vi "LHF.DB.Mongo.Bson.ToVariant.vi"(7 "type":variant, 8 "error in (no error)":errorcluster, 11 "BsonValue":refnum<k24>) -> (0 "error out":errorcluster, 2 "data":variant, 3 "BsonValue 2":refnum<k24>)   [LabVIEW 2013, in "LHF.DB.Mongo.lvclass"]
uses:
  LHF.DB.Mongo.lvclass
  C:/Users/Ricardo/Desktop/Projetos/LabVIEW-MongoDB/src/Driver/MongoDB.Bson.dll
  Driver/MongoDB.Bson.dll
  <vilib>/Utility/VariantDataType/VariantType.lvlib
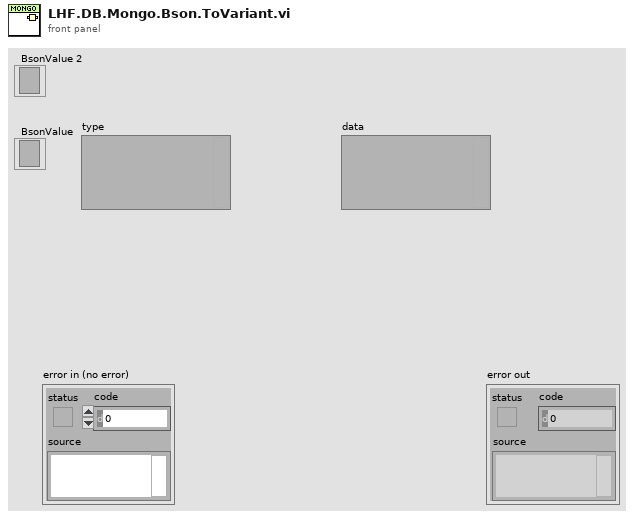
[diagram p1: front panel]
types:
  T1 = typedef "VariantType.lvlib/Type.ctl" = enum8{"Invalid Type", "Void", "I8", "I16", "I32", "I64", "U8", "U16", "U32", "U64", "Single Float", "Double Float", "Extended Float", "Single Complex", "Double Complex", "Extended Complex", "Enum U8", "Enum U16", "Enum U32", "Enum U64", "Single Float With Unit", "Double Float With Unit", "Extended Float With Unit", "Single Complex with Unit", "Double Complex with Unit", "Extended Complex with Unit", "Boolean", "String", "Path", "Picture", "Tag", "Array", "Cluster", "Variant", "LV Variant", "Waveform", "Timestamp", "Digital Waveform", "Digital Data", "ExpressData", "Refnum", "External Data", "VI", "Poly VI", "LabVIEW Class Instance", "Fixed Point"}
  T2 = typedef "LHF.DB.Mongo.lvclass/LHF.DB.Mongo.Typedef.VariantData.ctl" = cluster{"Type Enum":T1, "Name":string, "Variant":variant}
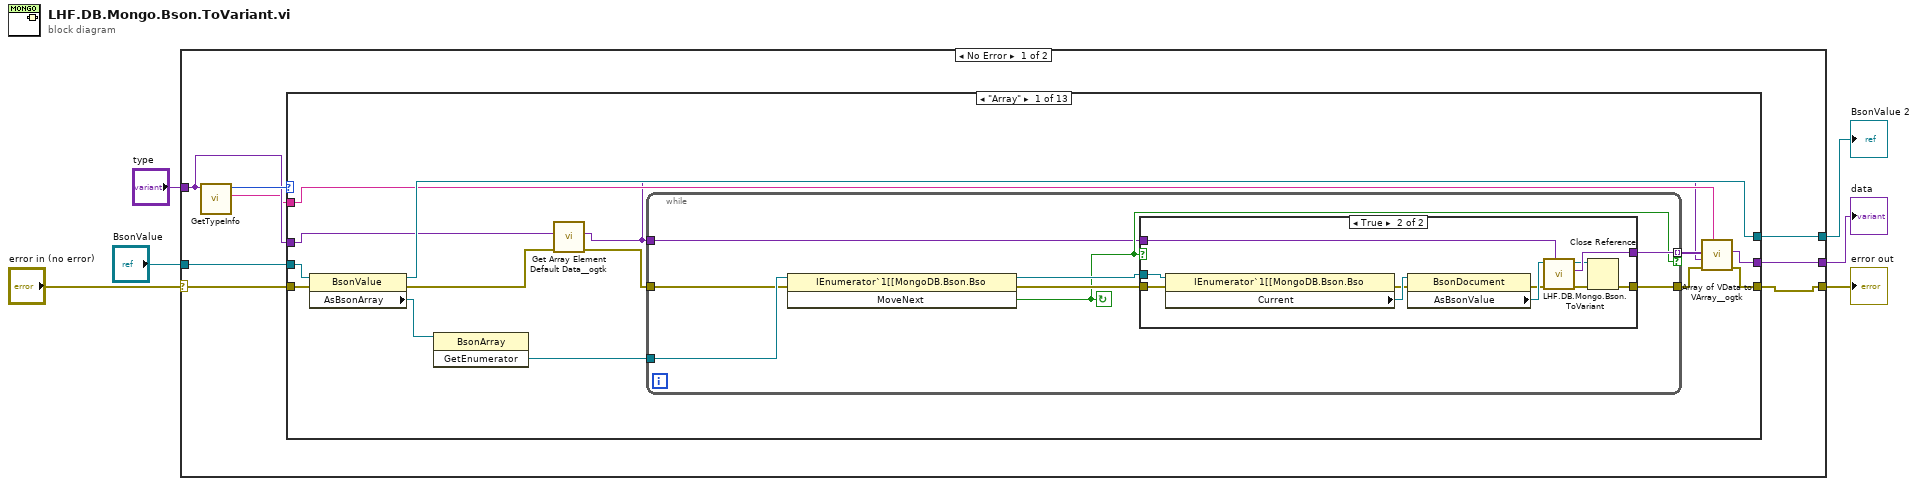
[diagram p0: block diagram]
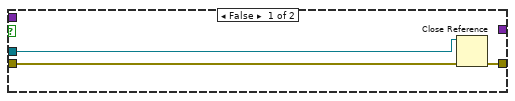
[diagram p2: hidden frame]
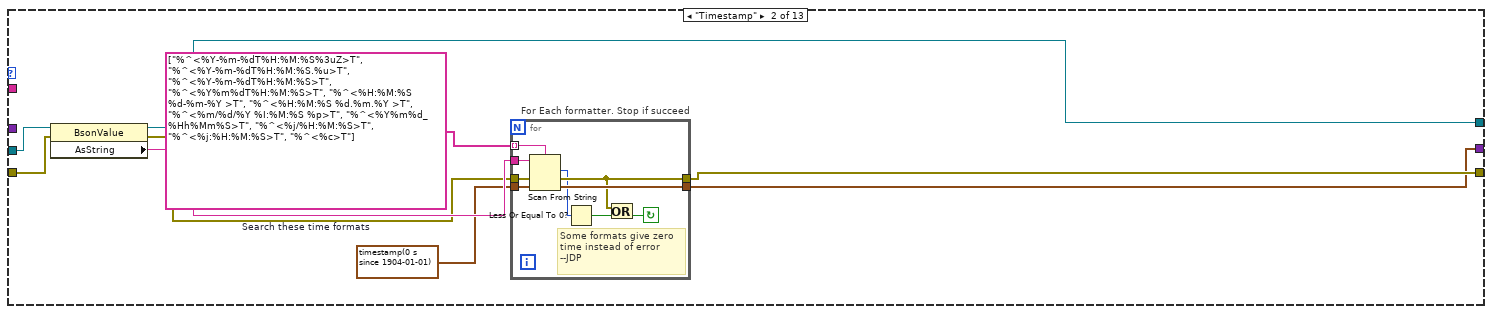
[diagram p3: hidden frame]
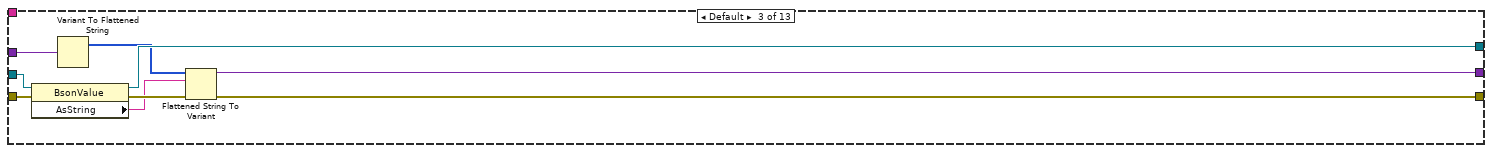
[diagram p4: hidden frame]
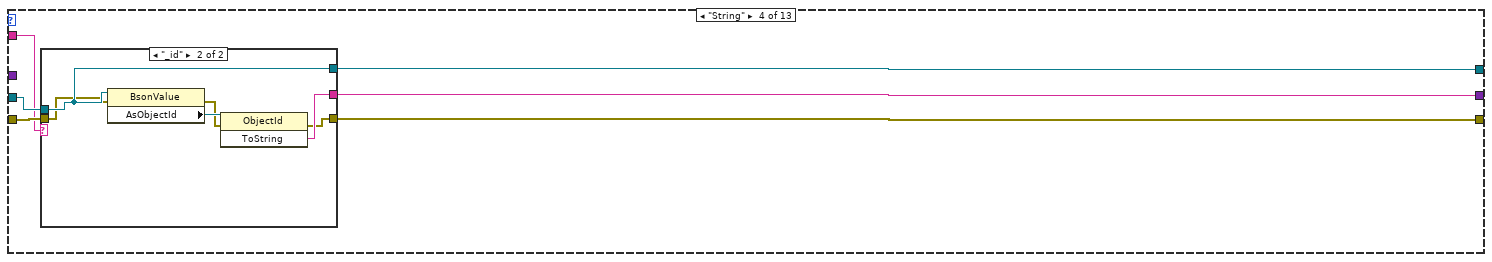
[diagram p5: hidden frame]
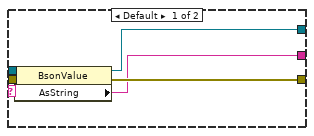
[diagram p6: hidden frame]
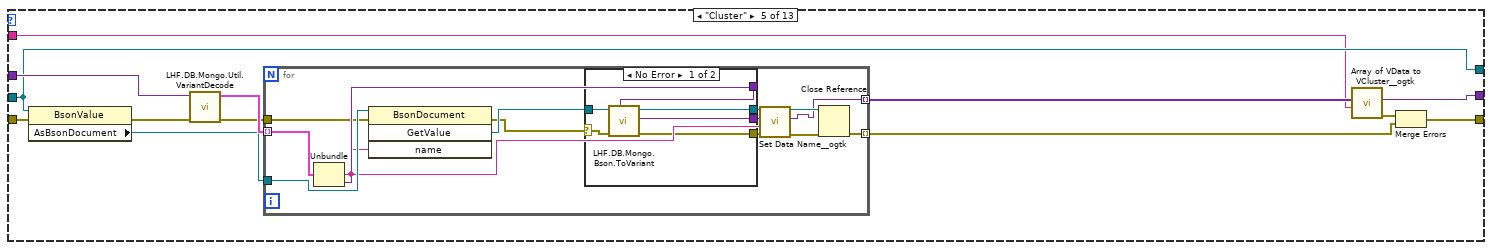
[diagram p7: hidden frame]
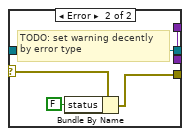
[diagram p8: hidden frame]
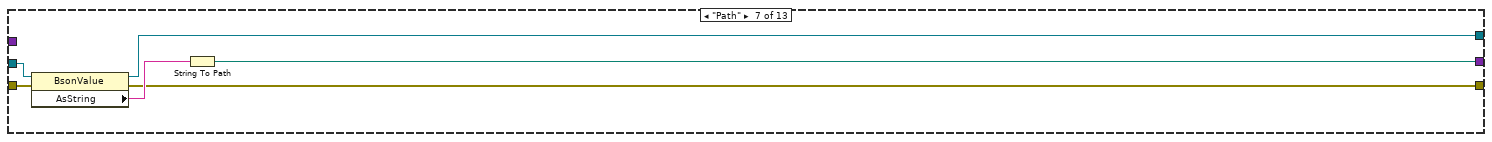
[diagram p10: hidden frame]
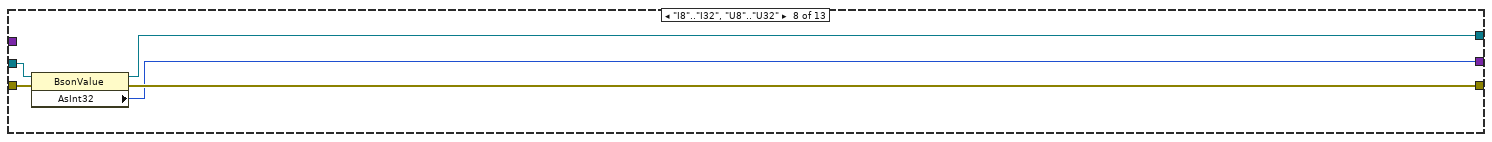
[diagram p11: hidden frame]
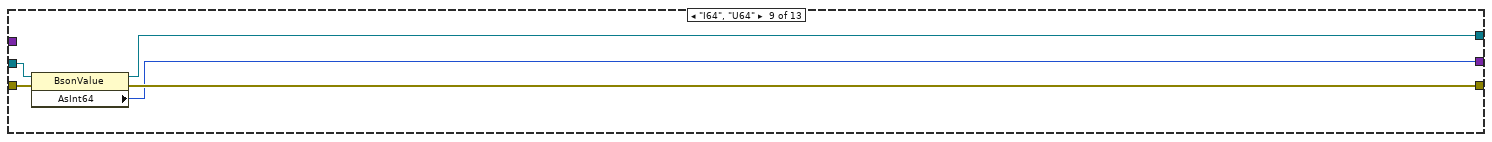
[diagram p12: hidden frame]
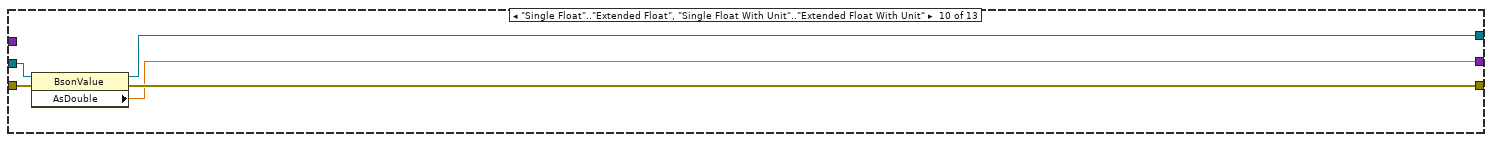
[diagram p13: hidden frame]
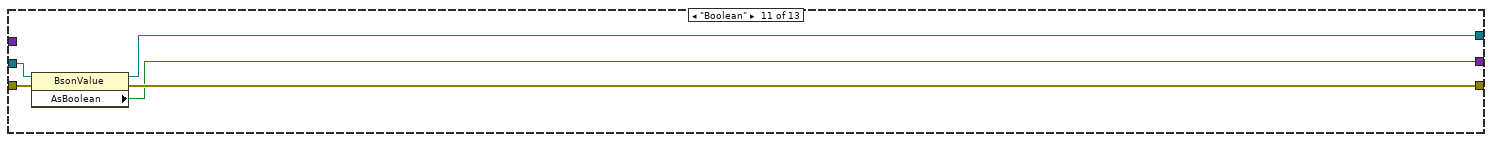
[diagram p14: hidden frame]
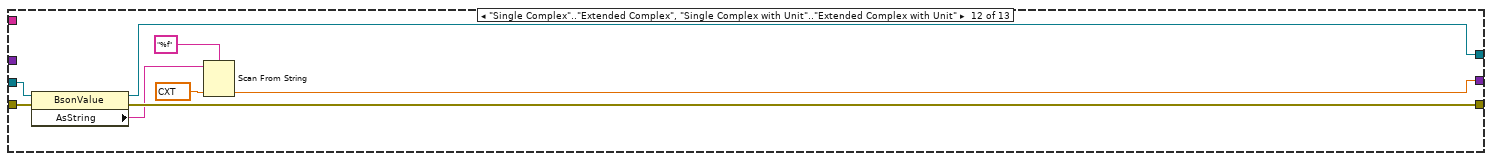
[diagram p15: hidden frame]
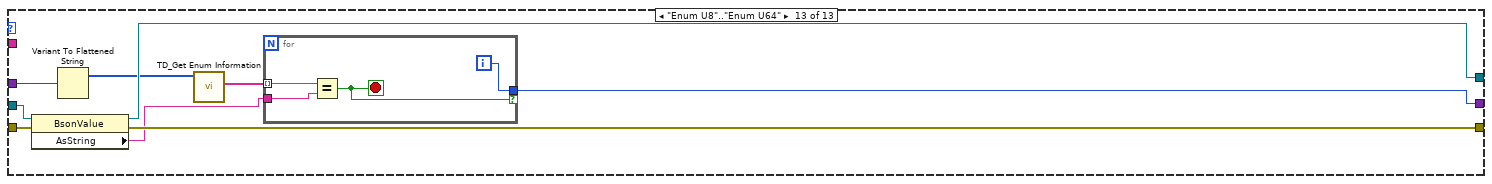
[diagram p16: hidden frame]
diagram:
  n1 = case shown="No Error" "error in (no error)" {
    selector: "error in (no error)" -> [w12 w183]
    tunnel: [w8 w183] -> w5
    tunnel: "BsonValue" -> [w14 w182]
    tunnel: "type" -> [w10 _]
    tunnel: [w13 w182] -> w2
    tunnel: [w7 _] -> w1
    frame No Error {
      n2 = call <vilib>:"GetTypeInfo.vi"("Variant"=w10) -> ("Name"=w9:string, "Type Enum"=w11:T1)  [unwired: 6 in, 3 out]
      n3 = case shown="\"Array\"" w11 {
        tunnel: w14 -> [w28 w58 w77 w83 w100 w133 w140 w145 w150 w155 w160 w168 w177]
        tunnel: [w26 w52 w75 w81 w100 w133 w136 w142 w147 w152 w157 w165 w174] -> w13
        tunnel: [w18 w51 w69 w79 w99 w134 w135 w141 w146 w151 w156 w162 w169] -> w7
        tunnel: w12 -> [w27 w54 w76 w82 w97 w132 w138 w144 w149 w154 w159 w167 w176]
        tunnel: [w15 w53 w71 w80 w103 w132 w137 w143 w148 w153 w158 w166 w175] -> w8
        tunnel: w10 -> [w23 _ w74 _ w107 w134 _ _ _ _ _ _ w173]
        tunnel: w9 -> [w17 _ _ w78 w95 _ _ _ _ _ _ _ _]
        frame "Array" {
          n4 = property class="BsonValue"(reference=w28, error in=w27) -> (reference out=w26:refnum<k24>, error out=w22:errorcluster, "AsBsonArray"=w25:refnum<k24>)
          n5 = invoke class="BsonArray" method="GetEnumerator"(reference=w25) -> ("GetEnumerator"=w24:refnum<k24>)  [unwired: 2 in, 2 out]
          n6 = call <userlib>:"Get Array Element Default Data__ogtk.vi"("error in (no error)"=w22, "Array"=w23) -> ("error out"=w21:errorcluster, "Array Element Default Data"=w16:variant)  [unwired: 8 in]
          n7 = while {
            tunnel: [w34] -> w19 mode=indexing if=w31
            tunnel: [w32] -> w20
            tunnel: w24 -> [w36]
            tunnel: w16 -> [w30]
            tunnel: w21 -> [w29]
            stop <- w31 continue-if-true
            n8 = invoke class="IEnumerator`1[[MongoDB.Bson.Bso" method="MoveNext"(reference=w36, error in=w29) -> (reference out=w35:refnum<k24>, error out=w33:errorcluster, "MoveNext"=w31:bool)  [unwired: 1 in]
            n9 = case shown="True" w31 {
              tunnel: w35 -> [w38 w50]
              tunnel: [_ w47] -> w34
              tunnel: w33 -> [w39 w49]
              tunnel: [w37 w48] -> w32
              tunnel: w30 -> [_ w46]
              frame False {
                n10 = Close Reference(reference=w38, error in (no error)=w39) -> (error out=w37:errorcluster)
              }
              frame True {
                n11 = property class="IEnumerator`1[[MongoDB.Bson.Bso"(reference=w50, error in=w49) -> (error out=w41:errorcluster, "Current"=w43:refnum<k24>)  [unwired: 1 out]
                n12 = property class="BsonDocument"(reference=w43, error in=w41) -> (error out=w40:errorcluster, "AsBsonValue"=w42:refnum<k24>)  [unwired: 1 out]
                n13 = call "LHF.DB.Mongo.Bson.ToVariant.vi"("type"=w46, "error in (no error)"=w40, "BsonValue"=w42) -> ("error out"=w44:errorcluster, "data"=w47:variant, "BsonValue 2"=w45:refnum<k24>)  [unwired: 6 in]
                n14 = Close Reference(reference=w45, error in (no error)=w44) -> (error out=w48:errorcluster)
              }
            }
          }
          n15 = call <userlib>:"Array of VData to VArray__ogtk.vi"("Array Name"=w17, "error in (no error)"=w20, "Element Type (when empty)"=w16, "1D Array of VData"=w19) -> ("error out"=w15:errorcluster, "VArray"=w18:variant)  [unwired: 6 in]
        }
        frame "Timestamp" {
          w59 = string[] ["%^<%Y-%m-%dT%H:%M:%S%3uZ>T", "%^<%Y-%m-%dT%H:%M:%S.%u>T", "%^<%Y-%m-%dT%H:%M:%S>T", "%^<%Y%m%dT%H:%M:%S>T", "%^<%H:%M:%S %d-%m-%Y >T", "%^<%H:%M:%S %d.%m.%Y >T", "%^<%m/%d/%Y %I:%M:%S %p>T", "%^<%Y%m%d_%Hh%Mm%S>T", "%^<%j/%H:%M:%S>T", "%^<%j:%H:%M:%S>T", "%^<%c>T"]  # Search these time formats
          n16 = property class="BsonValue"(reference=w58, error in=w54) -> (reference out=w52:refnum<k24>, error out=w55:errorcluster, "AsString"=w57:string)
          n17 = for "For Each formatter. Stop if succeed" {
            tunnel: [w68] -> w51
            tunnel: w55 -> [w67]
            tunnel: [w61] -> w53
            tunnel: timestamp(0 s since 1904-01-01) ("default value 1") -> [w66]
            tunnel: w57 -> [w65]
            tunnel: w59 -> [w64] mode=indexing
            stop <- w62 continue-if-true
            # "Some formats give zero\ntime instead of error\n--JDP"
            n18 = Scan From String(format string=w64, input string=w65, error in=w67, default 1=w66) -> (offset past scan=w60:u32, error out=w61:errorcluster, output 1=w68:timestamp)  [unwired: 1 in, 1 out]
            n19 = Less Or Equal To 0?(x=w60) -> (x <= 0?=w63:bool)
            n20 = Or(x=w61, y=w63) -> (x .or. y?=w62:bool)
          }
        }
        frame Default {
          n21 = property class="BsonValue"(reference=w77, error in=w76) -> (reference out=w75:refnum<k24>, error out=w72:errorcluster, "AsString"=w70:string)
          n22 = Variant To Flattened String(Variant=w74) -> (1:w73:i16[])  [unwired: 1 out]
          n23 = Flattened String To Variant(4:w72, 6:w70, 7:w73) -> (0:w71:errorcluster, 3:w69:variant)
        }
        frame "String" {
          n24 = case shown="\"_id\"" w78 {
            tunnel: w83 -> [w88 w92]
            tunnel: w82 -> [w87 w89]
            tunnel: [w86 w92] -> w81
            tunnel: [w85 w91] -> w80
            tunnel: [w84 w93] -> w79
            frame Default {
              n25 = property class="BsonValue"(reference=w88, error in=w87) -> (reference out=w86:refnum<k24>, error out=w85:errorcluster, "AsString"=w84:string)
            }
            frame "_id" {
              n26 = property class="BsonValue"(reference=w92, error in=w89) -> (error out=w90:errorcluster, "AsObjectId"=w94:refnum<k24>)  [unwired: 1 out]
              n27 = invoke class="ObjectId" method="ToString"(reference=w94, error in=w90) -> (error out=w91:errorcluster, "ToString"=w93:string)  [unwired: 1 in, 1 out]
            }
          }
        }
        frame "Cluster" {
          n28 = property class="BsonValue"(reference=w100, error in=w97) -> (error out=w102:errorcluster, "AsBsonDocument"=w96:refnum<k24>)  [unwired: 1 out]
          n29 = call "LHF.DB.Mongo.Util.VariantDecode.vi"("error in (no error)"=w102, "variant"=w107) -> ("error out"=w101:errorcluster, "Variant Data"=w106:T2[])  [unwired: 7 in, 1 out]
          n30 = for {
            tunnel: w106 -> [w120] mode=indexing
            tunnel: w96 -> [w118]
            tunnel: [w110] -> w105 mode=indexing
            tunnel: [w116] -> w104 mode=indexing
            tunnel: w101 -> [w115]
            n31 = Unbundle(w120) -> ("Name"=w112:string, "Variant"=w119:variant)  [unwired: 1 out]
            n32 = invoke class="BsonDocument" method="GetValue"(reference=w118, error in=w115, "name"=w112) -> (error out=w108:errorcluster, "GetValue"=w114:refnum<k24>)  [unwired: 1 in, 2 out]
            n33 = case shown="No Error" w108 {
              selector: w108 -> [w121 w129]
              tunnel: w119 -> [w126 w131]
              tunnel: [w125 w130] -> w117
              tunnel: w114 -> [w124 w130]
              tunnel: [w123 w128] -> w113
              tunnel: [w122 w131] -> w111
              frame No Error {
                n34 = call "LHF.DB.Mongo.Bson.ToVariant.vi"("type"=w126, "error in (no error)"=w121, "BsonValue"=w124) -> ("error out"=w123:errorcluster, "data"=w122:variant, "BsonValue 2"=w125:refnum<k24>)  [unwired: 6 in]
              }
              frame Error {
                # "TODO: set warning decently\nby error type"
                n35 = Bundle By Name(cluster=w129, "status"=FALSE) -> (w128:errorcluster)
              }
            }
            n36 = call <userlib>:"Set Data Name__ogtk.vi"("error in (no error)"=w113, "Data Name"=w112, "Data"=w111) -> ("error out"=w109:errorcluster, "Renamed Data"=w110:variant)  [unwired: 7 in]
            n37 = Close Reference(reference=w117, error in (no error)=w109) -> (error out=w116:errorcluster)
          }
          n38 = call <userlib>:"Array of VData to VCluster__ogtk.vi"("Cluster Name"=w95, "Array"=w105) -> ("error out"=w98:errorcluster, "VCluster"=w99:variant)  [unwired: 8 in]
          n39 = Merge Errors(w98, w104) -> (w103:errorcluster)
        }
        frame "Void" {
        }
        frame "Path" {
          n40 = property class="BsonValue"(reference=w140, error in=w138) -> (reference out=w136:refnum<k24>, error out=w137:errorcluster, "AsString"=w139:string)
          n41 = String To Path(string=w139) -> (path=w135:path)
        }
        frame "I8".."I32", "U8".."U32" {
          n42 = property class="BsonValue"(reference=w145, error in=w144) -> (reference out=w142:refnum<k24>, error out=w143:errorcluster, "AsInt32"=w141:i32)
        }
        frame "I64", "U64" {
          n43 = property class="BsonValue"(reference=w150, error in=w149) -> (reference out=w147:refnum<k24>, error out=w148:errorcluster, "AsInt64"=w146:i64)
        }
        frame "Single Float".."Extended Float", "Single Float With Unit".."Extended Float With Unit" {
          n44 = property class="BsonValue"(reference=w155, error in=w154) -> (reference out=w152:refnum<k24>, error out=w153:errorcluster, "AsDouble"=w151:dbl)
        }
        frame "Boolean" {
          n45 = property class="BsonValue"(reference=w160, error in=w159) -> (reference out=w157:refnum<k24>, error out=w158:errorcluster, "AsBoolean"=w156:bool)
        }
        frame "Single Complex".."Extended Complex", "Single Complex with Unit".."Extended Complex with Unit" {
          n46 = property class="BsonValue"(reference=w168, error in=w167) -> (reference out=w165:refnum<k24>, error out=w166:errorcluster, "AsString"=w164:string)
          n47 = Scan From String(format string="%f", input string=w164, default 1=cxt 0.0+0.0i) -> (output 1=w162:cxt)  [unwired: 2 in, 3 out]
        }
        frame "Enum U8".."Enum U64" {
          n48 = property class="BsonValue"(reference=w177, error in=w176) -> (reference out=w174:refnum<k24>, error out=w175:errorcluster, "AsString"=w170:string)
          n49 = Variant To Flattened String(Variant=w173) -> (1:w172:i16[])  [unwired: 1 out]
          n50 = call <vilib>:"TD_Get Enum Information.vi"("Type descriptor"=w172) -> ("Value Names"=w171:string[])  [unwired: 9 in, 1 out]
          n51 = for {
            tunnel: w171 -> [w181] mode=indexing
            tunnel: w170 -> [w180]
            tunnel: [w179] -> w169 if=w178
            i -> [w179]
            stop <- w178 stop-if-true
            n52 = Equal?(x=w181, y=w180) -> (x = y?=w178:bool)
          }
        }
      }
    }
    frame Error {
    }
  }
  "error out" <- w5
  "data" <- w1
  "BsonValue 2" <- w2
